vi "BW and No Fire Results to Table.vi"(7 "configuration file path":path, 8 "error in (no error)":errorcluster, 9 "No-Fire Result":bool, 10 "BW 2 Resistance":string, 11 "BW 1 Resistance":string) -> (0 "error out":errorcluster, 2 "Results Table":string[][](array[string]))   [LabVIEW 2018]
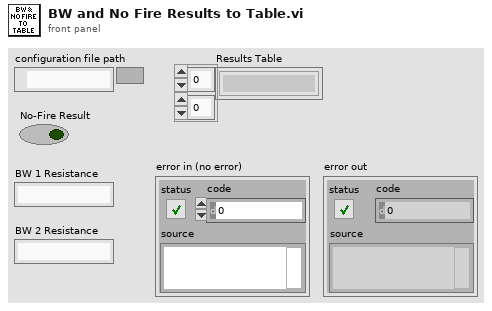
[diagram p1: front panel]
types:
  T1 = cluster{"BW1 Resistance (Ohms)":string, "BW2 Resistance (Ohms)":string, "BW1 No-Fire":string, "BW2 No-Fire":string, "BW1 Dielectric Strength (uA)":string, "BW2 Dielectric Strength (uA)":string, "BW1 Insulation Resistance (MOhms)":string, "BW2 Insulation Resistance (MOhms)":string}
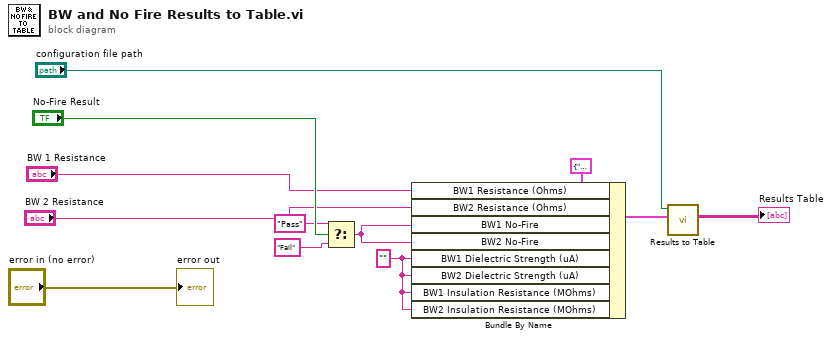
[diagram p0: block diagram]
diagram:
  w1 = "" ("BW1 Dielectric Strength (uA)")
  n1 = Select(t="Pass" ("BW1 Dielectric Strength (uA)"), s="No-Fire Result", f="Fail" ("BW1 Dielectric Strength (uA)")) -> (s? t:f=w8:string)
  n2 = Bundle By Name(cluster=T1 {"BW1 Resistance (Ohms)"="4870 ", "BW2 Resistance (Ohms)"="4870 ", "BW1 No-Fire"="4870 ", "BW2 No-Fire"="4870 ", "BW1 Dielectric Strength (uA)"="4870 ", "BW2 Dielectric Strength (uA)"="4870 ", "BW1 Insulation Resistance (MOhms)"="4870 ", "BW2 Insulation Resistance (MOhms)"="4870 "} ("Test Results"), "BW1 Resistance (Ohms)"="BW 1 Resistance", "BW2 Resistance (Ohms)"="BW 2 Resistance", "BW1 No-Fire"=w8, "BW2 No-Fire"=w8, "BW1 Dielectric Strength (uA)"=w1, "BW2 Dielectric Strength (uA)"=w1, "BW1 Insulation Resistance (MOhms)"=w1, "BW2 Insulation Resistance (MOhms)"=w1) -> (w3:T1)
  n3 = call "Results to Table.vi"("Test Results"=w3, "configuration file path"="configuration file path") -> ("Results Table"=→"Results Table":string[][])  [unwired: 8 in, 1 out]
  "error out" <- "error in (no error)"
